vi "Generate Firmware Libraries.vi"() -> ()   [LabVIEW 2011, in "LVH-LINX.lvlib"]
uses:
  vi.lib/LabVIEW Hacker/LINX/LVH-LINX.lvlib
  <vilib>/LabVIEW Hacker/LVH-Toolbox/Common/LVH-Common.lvlib
panel:
  out "Error Out":errorcluster
  in  "Libraries Destination Directory":path=path "C:/Users/samkristoff/Documents/Arduino/libraries"
  in  "Cancel Button":bool
  in  "Generate Button":bool
  # "This wizard will copy the LINX firmware source libraries into the directory specified below.\n\nDefault libraries locations:\nArduino IDE      C:\\Users\\<username>\\Documents\\Arduino\\libraries\nMPIDE                C:\\Users\\<username>\\Documents\\mpide\\libraries"
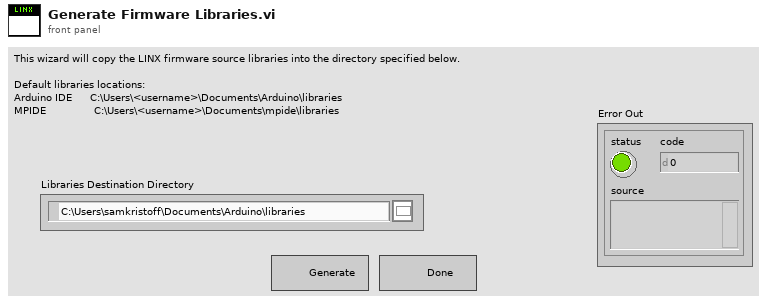
[diagram p1: front panel]
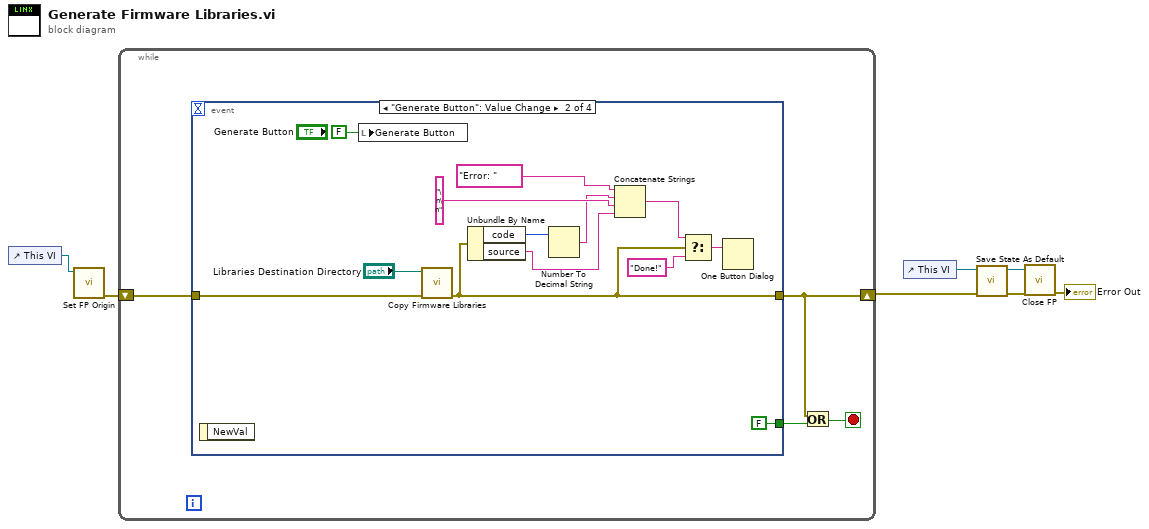
[diagram p0: block diagram]
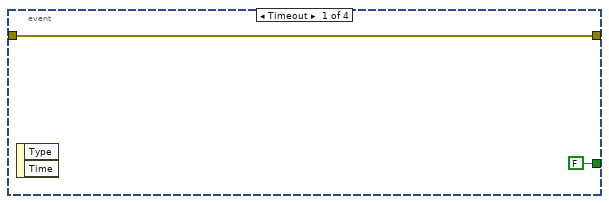
[diagram p2: hidden frame]
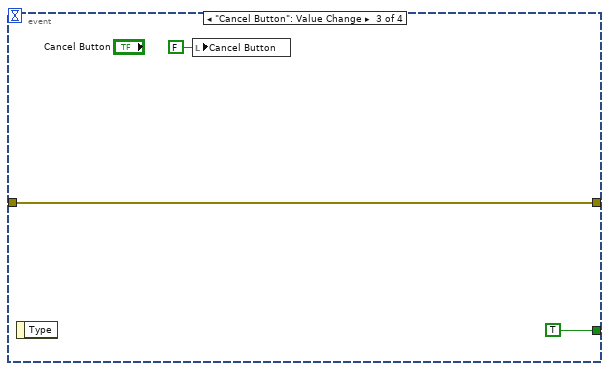
[diagram p3: hidden frame]
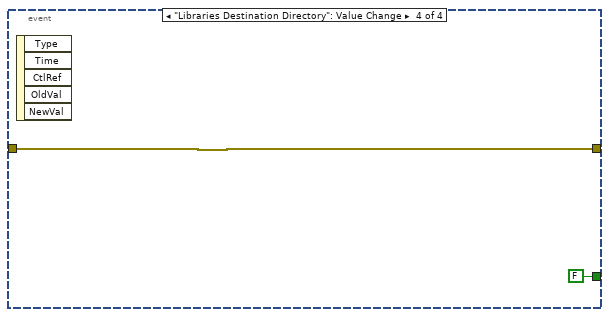
[diagram p4: hidden frame]
diagram:
  n1 = control-ref of="This VI"() -> (w7:refnum<vi>)
  n2 = call <vilib>:"Set FP Origin.vi"("VI Ref"=w7) -> ("Error Out"=w6:errorcluster)  [unwired: 10 in]
  n3 = while {
    shift-right: [w8] -> w5
    shift-left: w6 -> [w11]
    stop <- w9 stop-if-true
    n4 = event shown="[1] \"Generate Button\": Value Change" {
      selector: _ -> [_ _ _ _]
      dyn-events: _ -> [_ _ _ _]
      timeout: _ -> [_ _ _ _]
      tunnel: w11 -> [w13 w25 w27 w30]
      tunnel: [FALSE ("Cancel Button") FALSE ("Cancel Button") TRUE ("Cancel Button") FALSE ("Cancel Button")] -> w10
      tunnel: [w13 w18 w27 w30] -> w8
      event Timeout {
        n5 = event-data() -> ()  [unwired: 1 in, 2 out]
      }
      event "Generate Button": Value Change {
        n6 = event-data() -> ()  [unwired: 1 in, 1 out]
        n7 = local write "Generate Button"(FALSE ("Generate Button")) -> ()
        n8 = call "Copy Firmware Libraries.vi"("Error In"=w25, "Library Destination Dir"="Libraries Destination Directory") -> ("Error Out"=w18:errorcluster)  [unwired: 9 in]
        n9 = Unbundle By Name(w18) -> ("code"=w22:i32, "source"=w17:string)
        n10 = Number To Decimal String(number=w22) -> (decimal integer string=w14:string)  [unwired: 1 in]
        n11 = Concatenate Strings("Error: " ("message"), w14, "\n\n" ("string"), w17) -> (w21:string)
        n12 = Select(t=w21, s=w18, f="Done!" ("message")) -> (s? t:f=w19:string)
        n13 = One Button Dialog(message=w19) -> ()  [unwired: 1 in, 1 out]
      }
      event "Cancel Button": Value Change {
        n14 = event-data() -> ()  [unwired: 1 in, 1 out]
        n15 = local write "Cancel Button"(FALSE ("Cancel Button")) -> ()
      }
      event "Libraries Destination Directory": Value Change {
        n16 = event-data() -> ()  [unwired: 1 in, 5 out]
      }
    }
    n17 = Or(x=w8, y=w10) -> (x .or. y?=w9:bool)
  }
  n18 = control-ref of="This VI"() -> (w4:refnum<vi>)
  n19 = call <vilib>:"Save State As Default.vi"("Error In"=w5, "Target VI"=w4) -> ("Error Out"=w2:errorcluster, "Target VI"=w3:refnum<vi>)  [unwired: 8 in]
  n20 = call <vilib>:"Close FP.vi"("Error In"=w2, "VI Ref"=w3) -> ("Error Out"=→"Error Out":errorcluster)  [unwired: 9 in]
